vi "State_Mach_Inc.vi"(0 "State_Trigger":bool, 1 "Next_State":dbl, 2 "Time_Limit  (ms)":i32, 3 "Time_Enable":bool, 4 "Current_State":dbl) -> (7 "State":dbl)   [LabVIEW 2015]
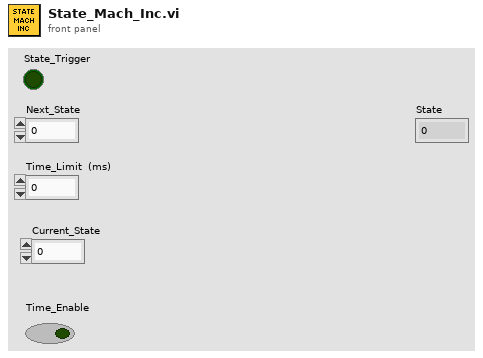
[diagram p1: front panel]
types:
  T1 = enum16{"Standard", "Momentary Falling", "Momentary Rising", "Momentary Falling and Rising"}
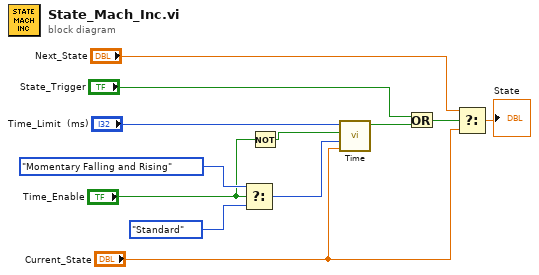
[diagram p0: block diagram]
diagram:
  n1 = Select(t=T1."Momentary Falling and Rising" ("Configuration"), s="Time_Enable", f=T1."Standard" ("Configuration")) -> (s? t:f=w4:T1)
  n2 = Not(x="Time_Enable") -> (.not. x?=w1:bool)
  n3 = call "Time.vi"("Reset_Int"="Current_State", "Configuration"=w4, "Reset"=w1, "Time_Limit  (ms)"="Time_Limit  (ms)") -> ("Time_Met"=w3:bool)  [unwired: 7 in]
  n4 = Or(x="State_Trigger", y=w3) -> (x .or. y?=w8:bool)
  n5 = Select(t="Next_State", s=w8, f="Current_State") -> (s? t:f=→"State":dbl)
